vi "Agilent E364X Series Output Dual Channel DC Volts.vi"(0 "VISA resource name":refnum<visa-resource-name>, 1 "Current Limit (0 Amps)":dbl format="%.2p", 2 "OVP Limit (22.0 Volts)":dbl=22.0 format="%.2p", 3 "OVP Enabled (True)":bool=TRUE, 5 "Output Enabled (False)":bool, 7 "Voltage Level (0.0 Volts)":dbl format="%.2p", 9 "Voltage Level 2 (0.0 Volts)":dbl format="%.2p", 11 "error in (no error)":errorcluster, 12 "Current Limit 2 (0 Amps)":dbl format="%.2p", 13 "OVP Limit 2 (22.0 Volts)":dbl=22.0 format="%.2p", 14 "OVP Enabled 2 (True)":bool=TRUE) -> ()   [LabVIEW 2013]
doc: "This VI configures the specifies power supply's channel to generate a DC voltage by taking the following steps:\n\n1) Configure current limit.\n\n2) Configure the over voltage protection.\n\n3) Configure the voltage level.\n\n4) Enable or disable the power output.\n\n5) Query the over voltage output state.\n\nNotes:\n\n(1) This VI takes a couple seconds to finish so that it may correctly get the current OVP value."
uses:
  <instrlib>/Agilent E364X Series/Agilent E364X Series.lvlib
panel:
  in  "Output Enabled 2 (False)":bool
  # "© 2005 National Instruments.  ALL RIGHTS RESERVED."
  # "Output 1"
  # "Output 2"
  # "For instructions,\nselect Show Context Help\nfrom the Help menu."
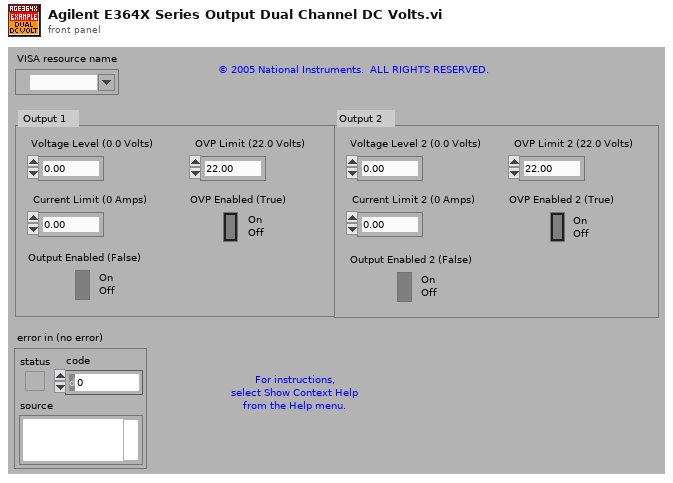
[diagram p1: front panel]
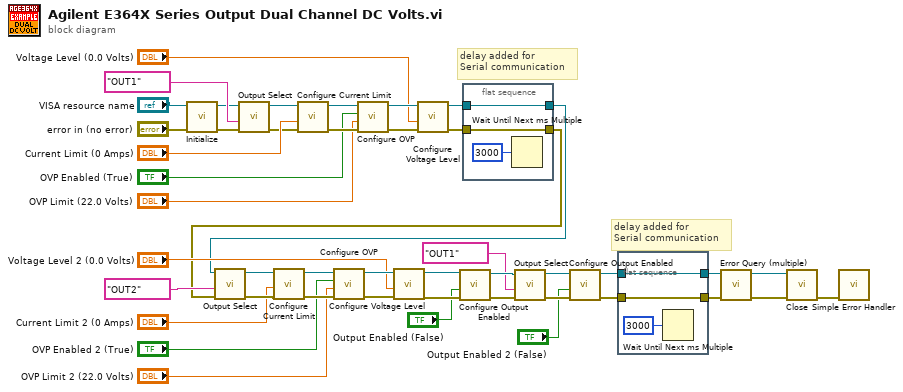
[diagram p0: block diagram]
diagram:
  # "delay added for \nSerial communication"
  # "delay added for \nSerial communication"
  n1 = call "Initialize.vi"("error in (no error)"="error in (no error)", "VISA resource name"="VISA resource name") -> ("error out"=w12:errorcluster, "VISA resource name out"=w13:refnum<visa-resource-name>)  [unwired: 8 in]
  n2 = call "Output Select.vi"("error in (no error)"=w2, "Instrument Select (Output 1)"="OUT2", "VISA resource name"=w1) -> ("error out"=w33:errorcluster, "VISA resource name out"=w34:refnum<visa-resource-name>)  [unwired: 7 in]
  n3 = call "Output Select.vi"("error in (no error)"=w12, "Instrument Select (Output 1)"="OUT1", "VISA resource name"=w13) -> ("error out"=w37:errorcluster, "VISA resource name out"=w38:refnum<visa-resource-name>)  [unwired: 7 in]
  n4 = call "Configure Current Limit.vi"("error in (no error)"=w33, "Current Limit (0.0 Amps)"="Current Limit 2 (0 Amps)", "VISA resource name"=w34) -> ("error out"=w31:errorcluster, "VISA resource name out"=w32:refnum<visa-resource-name>)  [unwired: 7 in]
  n5 = call "Configure Current Limit.vi"("error in (no error)"=w37, "Current Limit (0.0 Amps)"="Current Limit (0 Amps)", "VISA resource name"=w38) -> ("error out"=w46:errorcluster, "VISA resource name out"=w45:refnum<visa-resource-name>)  [unwired: 7 in]
  n6 = call "Configure OVP.vi"("error in (no error)"=w31, "Limit (22.0 Volts)"="OVP Limit 2 (22.0 Volts)", "OVP Enabled (T: On)"="OVP Enabled 2 (True)", "VISA resource name"=w32) -> ("error out"=w30:errorcluster, "VISA resource name out"=w29:refnum<visa-resource-name>)  [unwired: 6 in]
  n7 = call "Configure OVP.vi"("error in (no error)"=w46, "Limit (22.0 Volts)"="OVP Limit (22.0 Volts)", "OVP Enabled (T: On)"="OVP Enabled (True)", "VISA resource name"=w45) -> ("error out"=w42:errorcluster, "VISA resource name out"=w43:refnum<visa-resource-name>)  [unwired: 6 in]
  n8 = call "Configure Voltage Level.vi"("error in (no error)"=w30, "Level (0.0 Volts)"="Voltage Level 2 (0.0 Volts)", "VISA resource name"=w29) -> ("error out"=w23:errorcluster, "VISA resource name out"=w24:refnum<visa-resource-name>)  [unwired: 7 in]
  n9 = call "Configure Voltage Level.vi"("error in (no error)"=w42, "Level (0.0 Volts)"="Voltage Level (0.0 Volts)", "VISA resource name"=w43) -> ("error out"=w3:errorcluster, "VISA resource name out"=w4:refnum<visa-resource-name>)  [unwired: 7 in]
  n10 = call "Configure Output Enabled.vi"("error in (no error)"=w23, "Output Enabled (F: Off)"="Output Enabled (False)", "VISA resource name"=w24) -> ("error out"=w20:errorcluster, "VISA resource name out"=w22:refnum<visa-resource-name>)  [unwired: 7 in]
  n11 = flat-sequence {
    tunnel: w4 -> [w47]
    tunnel: [w48] -> w2
    tunnel: w3 -> [w48]
    tunnel: [w47] -> w1
    frame #0 {
      n12 = Wait Until Next ms Multiple(millisecond multiple=u32 3000) -> ()  [unwired: 1 out]
    }
  }
  n13 = call "Output Select.vi"("error in (no error)"=w20, "Instrument Select (Output 1)"="OUT1", "VISA resource name"=w22) -> ("error out"=w19:errorcluster, "VISA resource name out"=w21:refnum<visa-resource-name>)  [unwired: 7 in]
  n14 = call "Configure Output Enabled.vi"("error in (no error)"=w19, "Output Enabled (F: Off)"="Output Enabled 2 (False)", "VISA resource name"=w21) -> ("error out"=w5:errorcluster, "VISA resource name out"=w8:refnum<visa-resource-name>)  [unwired: 7 in]
  n15 = flat-sequence {
    tunnel: w8 -> [w51]
    tunnel: [w51] -> w7
    tunnel: [w50] -> w6
    tunnel: w5 -> [w50]
    frame #0 {
      n16 = Wait Until Next ms Multiple(millisecond multiple=u32 3000) -> ()  [unwired: 1 out]
    }
  }
  n17 = call "Error Query (multiple).vi"("error in (no error)"=w6, "VISA resource name"=w7) -> ("error out"=w10:errorcluster, "VISA resource name out"=w11:refnum<visa-resource-name>)  [unwired: 6 in, 2 out]
  n18 = call "Close.vi"("error in (no error)"=w10, "VISA resource name"=w11) -> ("error out"=w9:errorcluster)  [unwired: 9 in]
  n19 = call <vilib>:"Simple Error Handler.vi"("error in (no error)"=w9) -> ()  [unwired: 4 in, 5 out]
